vi "uA_Measurement_kit_v2.vi"() -> ()   [LabVIEW 2015]
uses:
  <vilib>/DAQmx/read.llb/DAQmx Read (Analog Wfm 1Chan NSamp).vi
  <vilib>/Utility/file.llb/Write Delimited Spreadsheet (string).vi
  <vilib>/measure/matone.llb/Extract Multiple Tone Information 1 Chan.vi
  <vilib>/DAQmx/miscellaneous.llb/DAQmx Fill In Error Info.vi
  <vilib>/measure/madcrms.llb/Basic Averaged DC-RMS for 1 Chan.vi
  <vilib>/measure/matone.llb/Extract Single Tone Information 1 Chan.vi
  <vilib>/measure/NI_MAPro.lvlib
  <vilib>/measure/NI_MABase.lvlib
panel:
  in  "uA_bank0":dbl=1.5 format="%#_13g"
  out "Task out":refnum<k21>="Stop"
  out "Sample rate":dbl=20000.0 format="%#_13g"
  out "Clear":bool=TRUE
  out "Ver":string
  out "seconds since 1Jan1904":timestamp
  out "error out":errorcluster
  in  "Tab Control":enum32{"Current Tracking", "Image", "CSV LOG"}(tab)
  out "uA_bank1":dbl
  in  "Calib":bool
  in  "Power ON/OFF":bool
  in  "Profile":enum16{"SAM", "DIANA", "Other..."}(ring)
  in  "Take Picture":bool
  in  "Orginal":bool
  in  "Clear Graph":bool
  out "Amp(Vdc)":dbl
  out "Freq(Hz)":dbl
  out "Waveform Graph 3":waveform(dbl)(graph)
  in  "ZOOM M1M2":bool
  in  "ZOOM -":bool
  in  "ZOOM +":bool
  in  "stop":bool
  out "VDUT- Vbat":dbl
  in  "Acquire Mode":enum16{"Streaming", "Read All", "Stop"}(ring)
  in  "Measure":bool
  in  "Current Range":T1(ring)
  out "Source":dbl
  in  "USB":tag="Dev1"
  out "Min value":dbl
  out "Max value":dbl
  out "Delta(s)":sgl
  in  "Center":bool
  out "Average":dbl
  in  "mA/uA":bool
  out "Waveform_main":waveform(sgl)(graph)
  out "Waveform_sub":waveform(dbl)(graph)
  out "Average (uA)":dbl
  in  "DUT Voltage Selector":enum16{"3.8VDC", "2.9VDC", "3.7VDC", "4.0VDC"}(ring)=enum."2.9VDC"
  in  "file List":i32(listbox)
  out "2D Picture":picture
  out "uA":dbl format="%#_4g"
  out "Vbat":dbl format="%#_4g"
  out "current time":timestamp
  in  "Record uA & Vbat":bool
  in  "Path":path
  out "uA":dbl(graph)
  out "Vbat Monitor":dbl(graph)
  # "uPower kit V2.1"
  # "Current"
  # "Voltage"
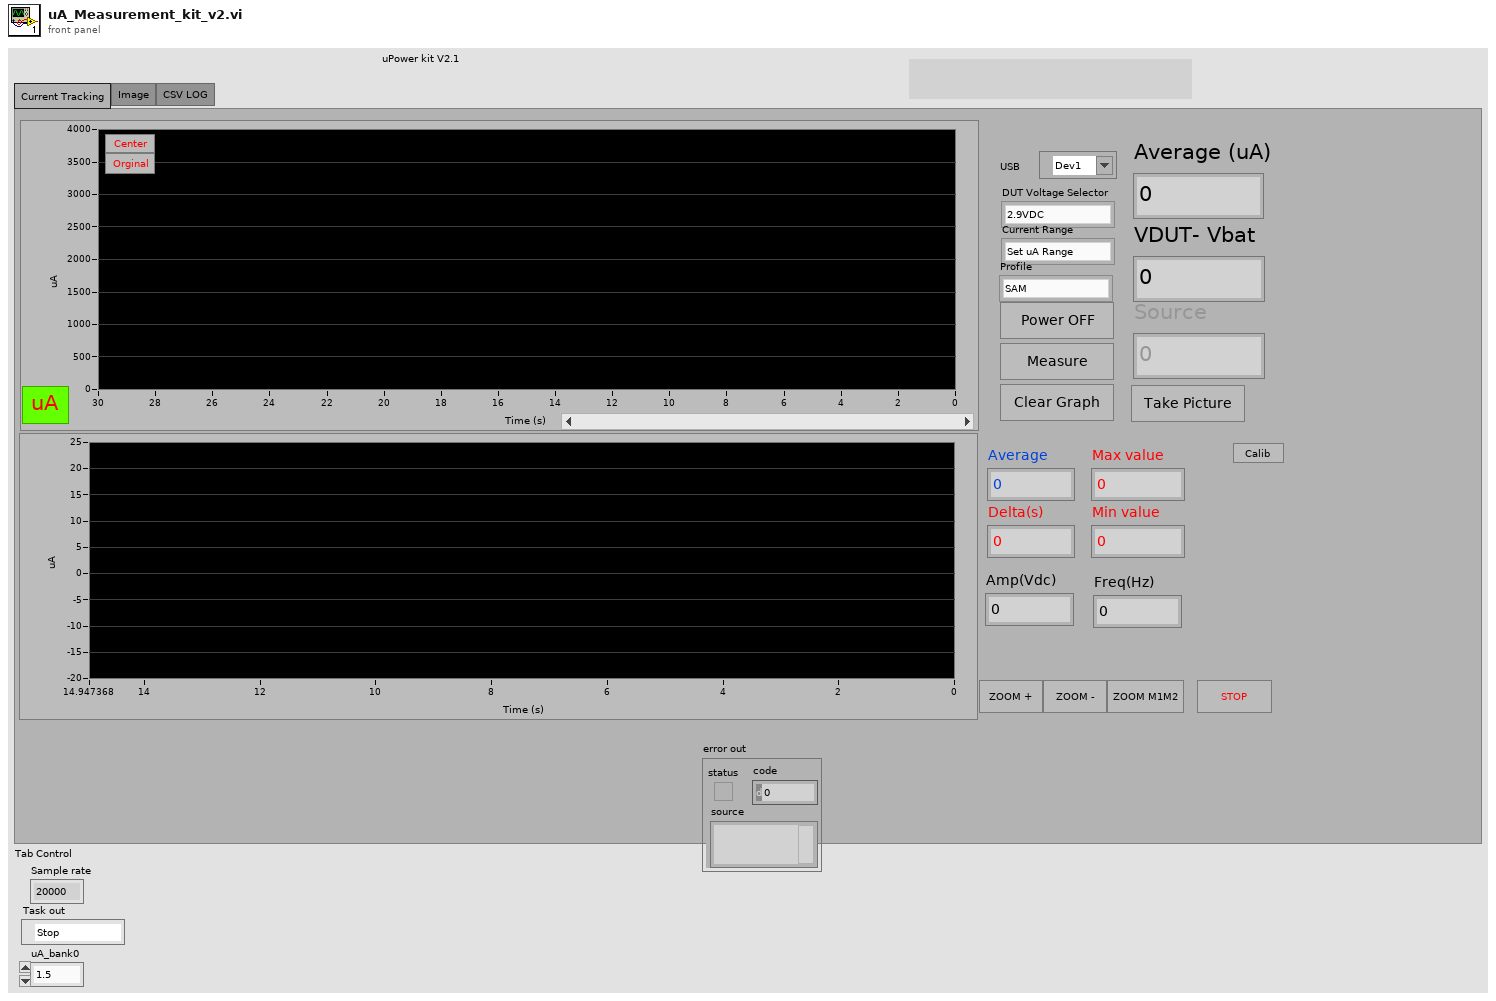
[diagram p1: front panel]
types:
  T1 = enum16{"Set uA Range ", "Set mA Range", "Measure Voltage"}
  T2 = typedef "LVCursorListTypeDef.ctl" = cluster{"Name":string, "Color":u32, "Style":u8, "Point Style":u8, "Name Visible":bool, "Allow Drag":bool, "Cursor Mode":u32, "Plot":i32, "Index":i32, "Position":cluster{"X":dbl, "Y":dbl}, "X Scale":u32, "Y Scale":u32, "Watch Plots":i32[], "Watch All Plots":bool, "Plot Area":i32, "Label Offset":cluster{"X":dbl, "Y":dbl}}[]
  T3 = typedef "imagedata.ctl" = cluster{"image type":i32, "image depth":i32, "image":u8[], "mask":u8[], "colors":u32[], "Rectangle":cluster{"left":i16, "top":i16, "right":i16, "bottom":i16}}
  T4 = enum32{"none", "input signal", "detected signal", "residual signal"}
  T5 = cluster{"detected frequency":dbl, "detected amplitude":dbl, "detected phase (deg)":dbl}[]
  T6 = cluster{"detected frequency":dbl, "detected amplitude":dbl, "detected phase (deg)":dbl}
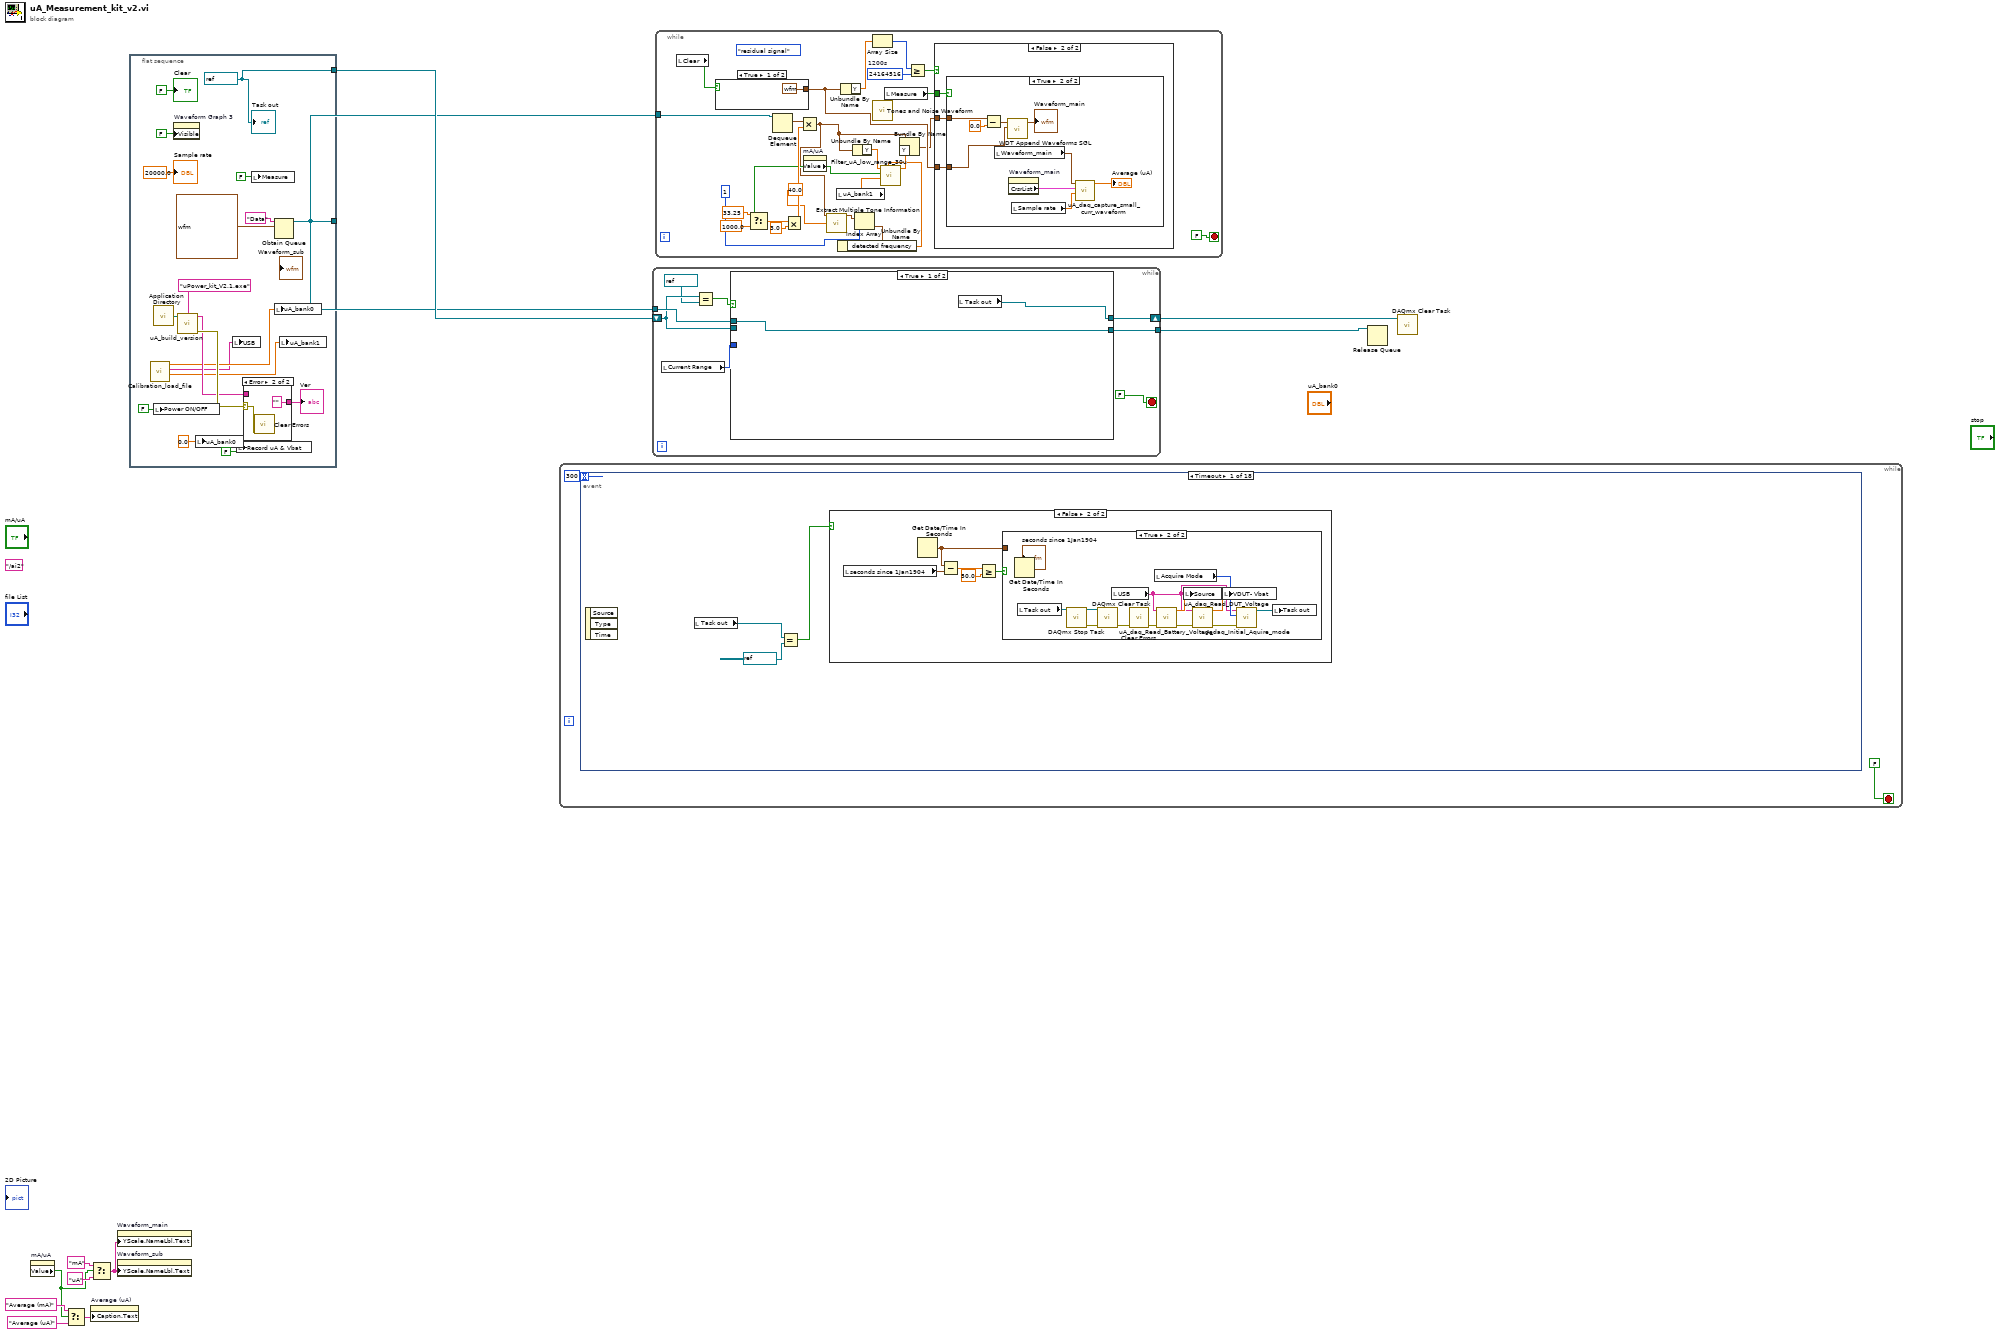
[diagram p0: block diagram]
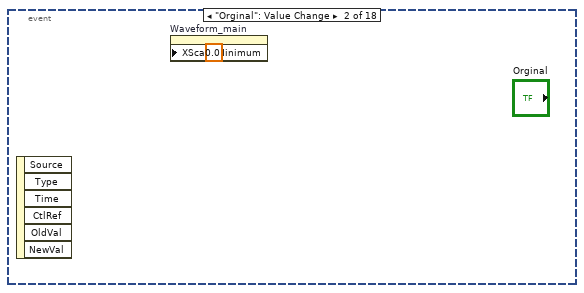
[diagram p5: hidden frame]
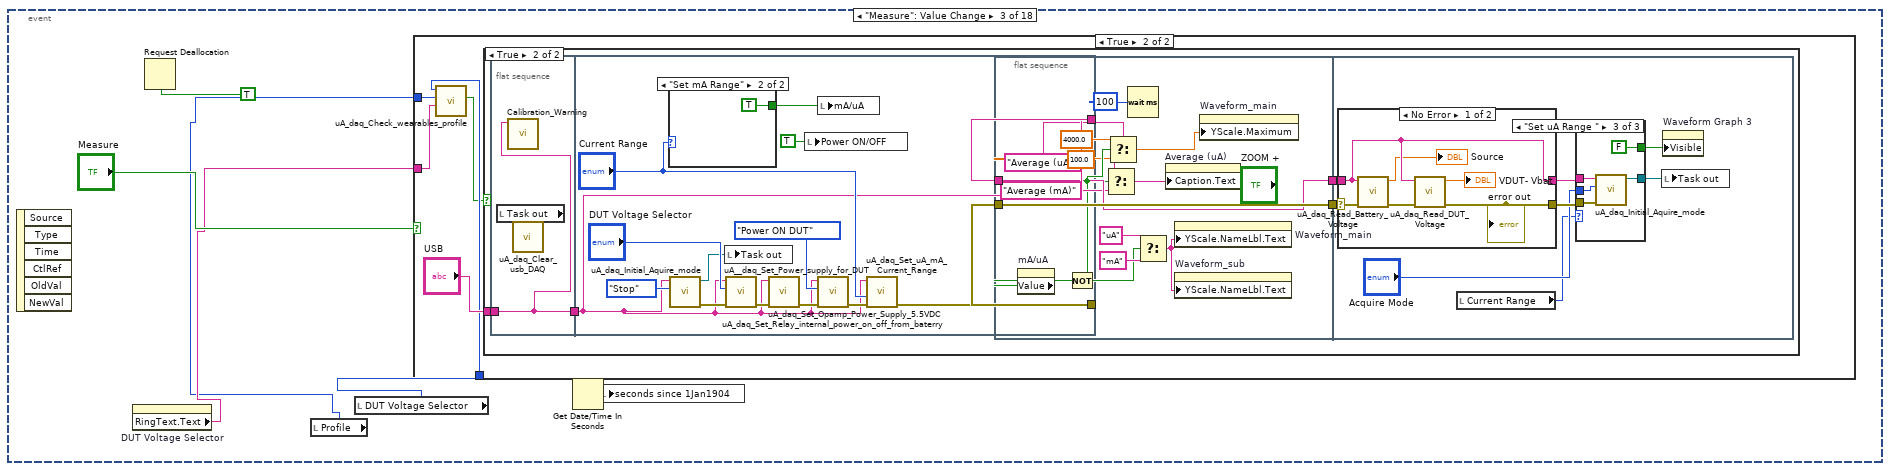
[diagram p6: hidden frame]
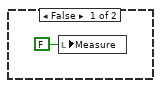
[diagram p8: hidden frame]
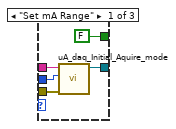
[diagram p9: hidden frame]
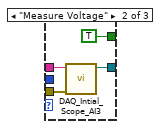
[diagram p10: hidden frame]
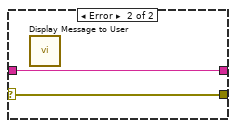
[diagram p11: hidden frame]
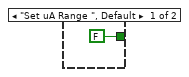
[diagram p12: hidden frame]
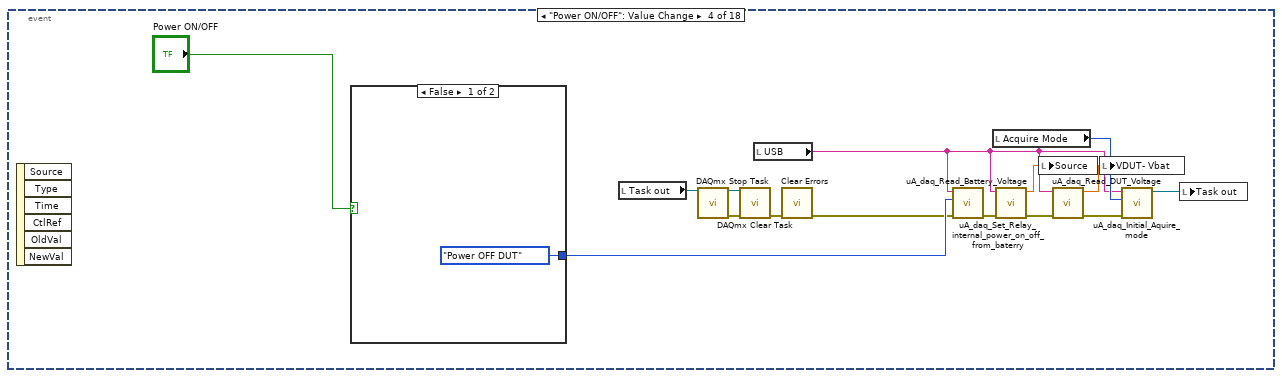
[diagram p13: hidden frame]
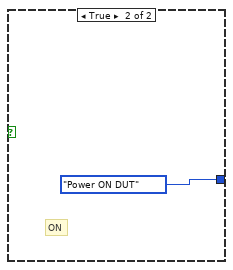
[diagram p14: hidden frame]
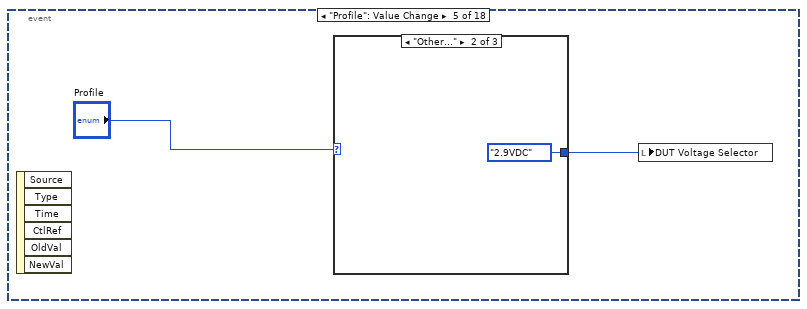
[diagram p15: hidden frame]
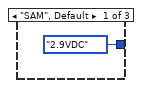
[diagram p16: hidden frame]
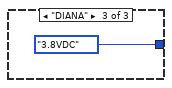
[diagram p17: hidden frame]
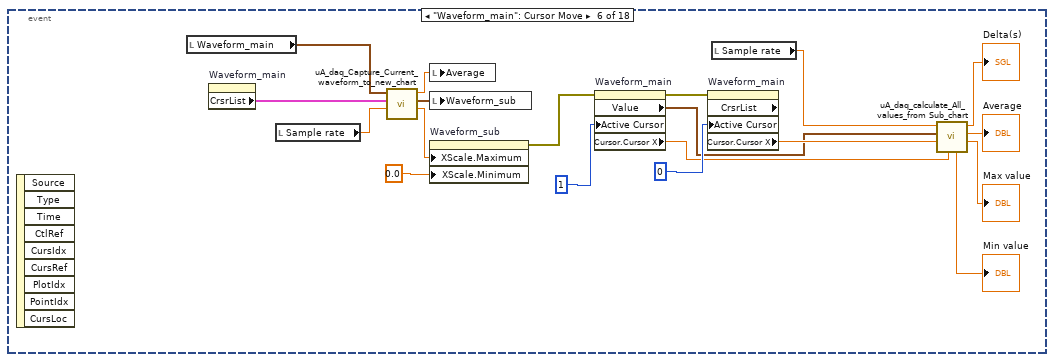
[diagram p18: hidden frame]
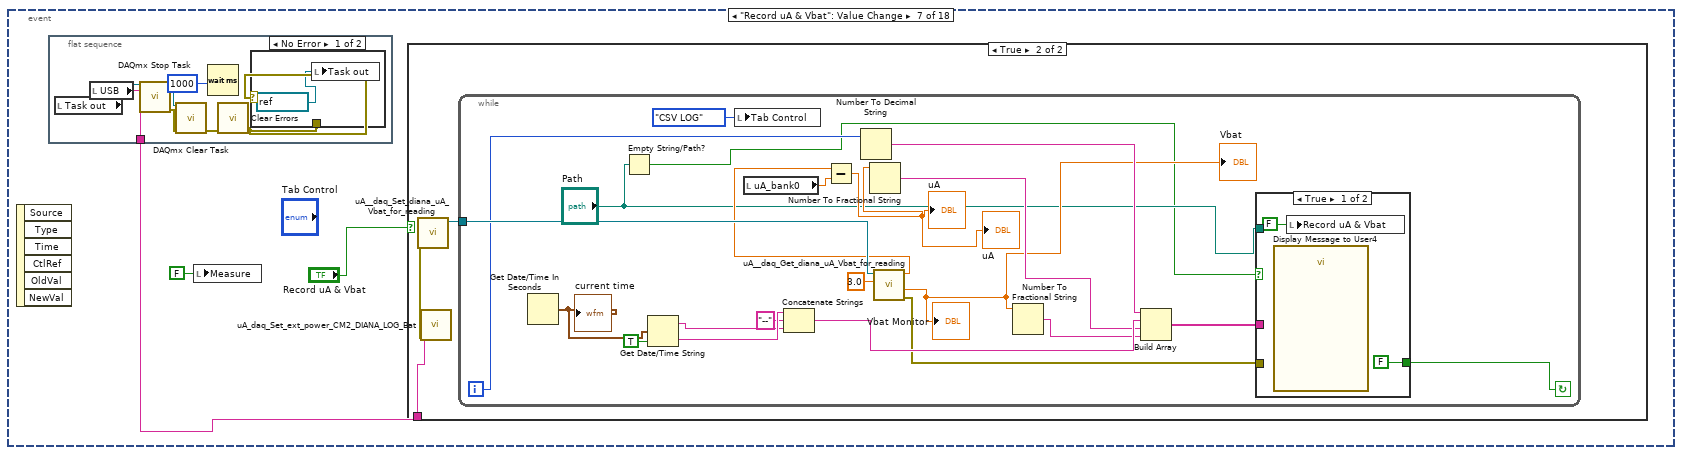
[diagram p19: hidden frame]
diagram:
  (unwired) "/ai2" ("string")
  n1 = property on="mA/uA" class="Bool (strict)"() -> ("Value"=w6:bool)  [unwired: 2 in, 2 out]
  n2 = Select(t="Average (mA)" ("Caption.Text"), s=w6, f="Average (uA)" ("Caption.Text")) -> (s? t:f=w4:string)
  n3 = property on="Average (uA)" class="DigNum (strict)"("Caption.Text"=w4) -> ()  [unwired: 2 in, 2 out]
  n4 = Select(t="mA" ("Caption.Text"), s=w6, f="uA" ("Caption.Text")) -> (s? t:f=w5:string)
  n5 = property on="Waveform_main" class="WFGraph (strict)"("YScale.NameLbl.Text"=w5) -> ()  [unwired: 2 in, 2 out]
  n6 = property on="Waveform_sub" class="WFGraph (strict)"("YScale.NameLbl.Text"=w5) -> ()  [unwired: 2 in, 2 out]
  n7 = flat-sequence {
    tunnel: [w22] -> w2
    tunnel: [w25] -> w1
    frame #0 {
      w22 = refnum<k21> "Stop" ("task out")
      n8 = call "Calibration_load_file.vi"() -> ("uABank1"=w15:dbl, "USB_DEV"=w14:string, "uABank0"=w16:dbl)  [unwired: 9 in]
      n9 = call <vilib>:"Application Directory.vi"() -> ("Application Directory"=w24:path)
      n10 = local write "Power ON/OFF"(FALSE ("Power ON/OFF")) -> ()
      n11 = property on="Waveform Graph 3" class="WFGraph (strict)"("Visible"=FALSE) -> ()  [unwired: 2 in, 2 out]
      n12 = call "uA_build_version.vi"("name or relative path"="uPower_kit_V2.1.exe", "path"=w24) -> ("error out"=w21:errorcluster, "FileVersion"=w20:string)  [unwired: 7 in, 1 out]
      n13 = local write "uA_bank0"(0.0 ("uA_calib_0")) -> ()
      n14 = local write "USB"(w14) -> ()
      n15 = local write "Record uA & Vbat"(FALSE ("Record uA & Vbat")) -> ()
      n16 = case shown="Error" w21 {
        selector: w21 -> [_ w33]
        tunnel: w20 -> [w31 _]
        tunnel: [w31 "" ("FileVersion")] -> w19
        frame No Error {
        }
        frame Error {
          n17 = call <vilib>:"Clear Errors.vi"("error in (no error)"=w33) -> ()  [unwired: 5 in, 2 out]
        }
      }
      "Ver" <- w19
      n18 = local write "Measure"(FALSE ("Measure")) -> ()
      n19 = Obtain Queue(name (unnamed)="Data", element data type=waveform(sgl) {"t0"=timestamp(0 s since 1904-01-01), "dt"=1.0, "Y"=[]} ("Waveform Chart 2")) -> (queue out=w25:refnum<queue>)  [unwired: 3 in, 2 out]
      n20 = local write "uA_bank0"(w16) -> ()
      n21 = local write "uA_bank1"(w15) -> ()
      "Clear" <- FALSE ("Clear")
      "Sample rate" <- 20000.0 ("Sample rate")
      "Task out" <- w22
    }
  }
  n22 = while {
    stop <- FALSE stop-if-true
    n23 = event shown="[0] Timeout" {
      selector: _ -> [_ _ _ _ _ _ _ _ _ _ _ _ _ _ _ _ _ _]
      dyn-events: _ -> [_ _ _ _ _ _ _ _ _ _ _ _ _ _ _ _ _ _]
      timeout: 300 -> [_ _ _ _ _ _ _ _ _ _ _ _ _ _ _ _ _ _]
      event Timeout {
        n24 = event-data() -> ()  [unwired: 1 in, 3 out]
        n25 = local read "Task out"() -> (w36:refnum<k21>)
        n26 = Equal?(x=w36, y=refnum<k21> "Stop") -> (x = y?=w37:bool)
        n27 = case shown="False" w37 {
          frame True {
          }
          frame False {
            n28 = local read "seconds since 1Jan1904"() -> (w39:timestamp)
            n29 = Get Date/Time In Seconds() -> (seconds since 1Jan1904=w40:timestamp)
            n30 = Subtract(x=w40, y=w39) -> (x-y=w43:dbl)
            n31 = Greater Or Equal?(x=w43, y=50.0) -> (x >= y?=w41:bool)
            n32 = case shown="True" w41 {
              tunnel: w40 -> [_ _]
              frame False {
              }
              frame True {
                n33 = Get Date/Time In Seconds() -> (seconds since 1Jan1904=→"seconds since 1Jan1904":timestamp)
                n34 = local read "Task out"() -> (w53:refnum<k21>)
                n35 = call <vilib>:"DAQmx Stop Task.vi"("task/channels in"=w53) -> ("task out"=w52:refnum<k21>, "error out"=w55:errorcluster)  [unwired: 13 in]
                n36 = call <vilib>:"DAQmx Clear Task.vi"("task in"=w52, "error in"=w55) -> ("error out"=w54:errorcluster)  [unwired: 13 in]
                n37 = local read "USB"() -> (w46:tag)
                n38 = call <vilib>:"Clear Errors.vi"("error in (no error)"=w54) -> ("error out"=w51:errorcluster)  [unwired: 5 in, 1 out]
                n39 = local read "Acquire Mode"() -> (w47:enum16{"Streaming", "Read All", "Stop"})
                n40 = call "uA_daq_Read_Battery_Voltage.vi"("error in"=w51, "USB DAQ"=w46) -> ("error out"=w48:errorcluster, "Battery_Voltage"=w50:dbl)  [unwired: 8 in]
                n41 = local write "Source"(w50) -> ()
                n42 = call "uA_daq_Read_DUT_Voltage.vi"("error in"=w48, "USB DAQ"=w46) -> ("error out"=w45:errorcluster, "DUT_Voltage"=w49:dbl)  [unwired: 8 in]
                n43 = local write "VDUT- Vbat"(w49) -> ()
                n44 = call "uA_daq_Initial_Aquire_mode.vi"("error in"=w45, "Acquire Mode"=w47, "USB DAQ"=w46) -> ("Refnum out"=w44:refnum<k21>)  [unwired: 7 in, 1 out]
                n45 = local write "Task out"(w44) -> ()
              }
            }
          }
        }
      }
      event "Orginal": Value Change {
        n46 = event-data() -> ()  [unwired: 1 in, 6 out]
        n47 = property on="Waveform_main" class="WFGraph (strict)"("XScale.Minimum"=0.0 ("X Scale.Range:Minimum")) -> ()  [unwired: 2 in, 2 out]
      }
      event "Measure": Value Change {
        n48 = event-data() -> ()  [unwired: 1 in, 6 out]
        n49 = property on="DUT Voltage Selector" class="Enum (strict)"() -> ("RingText.Text"=w60:string)  [unwired: 2 in, 2 out]
        n50 = Request Deallocation(TRUE ("flag")) -> ()
        n51 = local read "Profile"() -> (w58:enum16{"SAM", "DIANA", "Other..."})
        n52 = local read "DUT Voltage Selector"() -> (w59:enum16{"3.8VDC", "2.9VDC", "3.7VDC", "4.0VDC"})
        n53 = case shown="True" "Measure" {
          tunnel: w60 -> [_ w67]
          tunnel: w59 -> [_ w66]
          tunnel: w58 -> [_ w65]
          frame False {
          }
          frame True {
            n54 = call "uA_daq_Check_wearables_profile.vi"("VDUT"=w67, "Profile"=w65, "DUT Voltage Selector"=w66) -> ("Profile"=w64:bool)  [unwired: 7 in, 1 out]
            n55 = case shown="True" w64 {
              tunnel: "USB" -> [_ w71]
              frame False {
                n56 = local write "Measure"(FALSE ("Measure")) -> ()
              }
              frame True {
                n57 = flat-sequence {
                  tunnel: w71 -> [w120]
                  tunnel: [w120] -> w75
                  tunnel: [w129] -> w72
                  tunnel: [w123] -> w70
                  tunnel: w75 -> [w123]
                  frame #0 {
                    n58 = local read "Task out"() -> (w121:refnum<k21>)
                    n59 = call "Calibration_Warning.vi"("USB"=w120) -> ()  [unwired: 11 in]
                    n60 = call "uA_daq_Clear_usb_DAQ.vi"("Refnum in"=w121) -> ()  [unwired: 11 in]
                  }
                  frame #1 {
                    n61 = case shown="\"Set mA Range\"" "Current Range" {
                      tunnel: [FALSE ("mA/uA") TRUE ("mA/uA")] -> w127
                      frame "Set uA Range ", Default {
                      }
                      frame "Set mA Range" {
                      }
                    }
                    n62 = call "uA_daq_Initial_Aquire_mode.vi"("Acquire Mode"=enum16{"Streaming", "Read All", "Stop"}."Stop", "USB DAQ"=w123) -> ("error out"=w124:errorcluster, "Refnum out"=w125:refnum<k21>)  [unwired: 8 in]
                    n63 = local write "Task out"(w125) -> ()
                    n64 = call "uA__daq_Set_Power_supply_for_DUT.vi"("error in"=w124, "DUT Voltage Selector"="DUT Voltage Selector", "USB DAQ"=w123) -> ("error out"=w133:errorcluster)  [unwired: 8 in]
                    n65 = call "uA_daq_Set_Opamp_Power_Supply_5.5VDC.vi"("error in"=w133, "USB DAQ"=w123) -> ("error out"=w131:errorcluster)  [unwired: 9 in]
                    n66 = local write "Power ON/OFF"(TRUE ("Power ON/OFF")) -> ()
                    n67 = local write "mA/uA"(w127) -> ()
                    n68 = call "uA_daq_Set_Relay_internal_power_on_off_from_baterry.vi"("error in"=w131, "Power ON/OFF DUT"=enum16{"Power ON DUT", "Power OFF DUT"}."Power ON DUT", "USB DAQ"=w123) -> ("error out"=w130:errorcluster)  [unwired: 8 in]
                    n69 = call "uA_daq_Set_uA_mA_Current_Range.vi"("error in"=w130, "Current Range"="Current Range", "device name"=w123) -> ("error out"=w129:errorcluster)  [unwired: 8 in]
                  }
                }
                n70 = flat-sequence {
                  tunnel: w70 -> [w88]
                  tunnel: w72 -> [w89]
                  tunnel: [w89] -> w74
                  tunnel: [w88] -> w73
                  tunnel: w74 -> [w97]
                  tunnel: w73 -> [w96]
                  frame #0 {
                    n71 = property on="mA/uA" class="Bool (strict)"() -> ("Value"=w80:bool)  [unwired: 2 in, 2 out]
                    n72 = Not(x=w80) -> (.not. x?=w79:bool)
                    n73 = Select(t="Average (uA)" ("Caption.Text"), s=w79, f="Average (mA)" ("Caption.Text")) -> (s? t:f=w86:string)
                    n74 = Select(t=4000.0, s=w79, f=100.0) -> (s? t:f=w78:dbl)
                    n75 = Wait (ms)(milliseconds to wait=u32 100) -> ()  [unwired: 1 out]
                    n76 = Select(t="uA" ("Caption.Text"), s=w79, f="mA" ("Caption.Text")) -> (s? t:f=w81:string)
                    n77 = property on="Average (uA)" class="DigNum (strict)"("Caption.Text"=w86) -> ()  [unwired: 2 in, 2 out]
                    n78 = property on="Waveform_main" class="WFGraph (strict)"("YScale.NameLbl.Text"=w81) -> ()  [unwired: 2 in, 2 out]
                    n79 = property on="Waveform_sub" class="WFGraph (strict)"("YScale.NameLbl.Text"=w81) -> ()  [unwired: 2 in, 2 out]
                    n80 = property on="Waveform_main" class="WFGraph (strict)"("YScale.Maximum"=w78) -> ()  [unwired: 2 in, 2 out]
                  }
                  frame #1 {
                    n81 = case shown="No Error" w97 {
                      selector: w97 -> [w115 w119]
                      tunnel: w96 -> [w113 w118]
                      tunnel: [w114 w119] -> w95
                      tunnel: [w113 w118] -> w94
                      frame No Error {
                        n82 = call "uA_daq_Read_Battery_Voltage.vi"("error in"=w115, "USB DAQ"=w113) -> ("error out"=w117:errorcluster, "Battery_Voltage"=→"Source":dbl)  [unwired: 8 in]
                        n83 = call "uA_daq_Read_DUT_Voltage.vi"("error in"=w117, "USB DAQ"=w113) -> ("error out"=w114:errorcluster, "DUT_Voltage"=→"VDUT- Vbat":dbl)  [unwired: 8 in]
                        "error out" <- w114
                      }
                      frame Error {
                        n84 = call "Display Message to User"() -> ()  [unwired: 10 in, 2 out]
                      }
                    }
                    n85 = local read "Current Range"() -> (w91:T1)
                    n86 = case shown="\"Set uA Range \"" w91 {
                      tunnel: w95 -> [w102 w104 w111]
                      tunnel: w94 -> [w101 w106 w110]
                      tunnel: [w100 w105 w109] -> w93
                      tunnel: "Acquire Mode" -> [w99 _ w108]
                      tunnel: [FALSE ("Visible") TRUE ("Visible") FALSE ("Visible")] -> w90
                      frame "Set mA Range" {
                        n87 = call "uA_daq_Initial_Aquire_mode.vi"("error in"=w102, "Acquire Mode"=w99, "USB DAQ"=w101) -> ("Refnum out"=w100:refnum<k21>)  [unwired: 7 in, 1 out]
                      }
                      frame "Measure Voltage" {
                        n88 = call "DAQ_Intial_Scope_AI3.vi"("error in"=w104, "physical channel"=w106) -> ("task out"=w105:refnum<k21>)  [unwired: 8 in, 1 out]
                      }
                      frame "Set uA Range " {
                        n89 = call "uA_daq_Initial_Aquire_mode.vi"("error in"=w111, "Acquire Mode"=w108, "USB DAQ"=w110) -> ("Refnum out"=w109:refnum<k21>)  [unwired: 7 in, 1 out]
                      }
                    }
                    n90 = local write "Task out"(w93) -> ()
                    n91 = property on="Waveform Graph 3" class="WFGraph (strict)"("Visible"=w90) -> ()  [unwired: 2 in, 2 out]
                  }
                }
              }
            }
          }
        }
        n92 = Get Date/Time In Seconds() -> (seconds since 1Jan1904=w62:timestamp)
        n93 = local write "seconds since 1Jan1904"(w62) -> ()
      }
      event "Power ON/OFF": Value Change {
        n94 = event-data() -> ()  [unwired: 1 in, 6 out]
        n95 = case shown="False" "Power ON/OFF" {
          tunnel: [enum16{"Power ON DUT", "Power OFF DUT"}."Power OFF DUT" ("Power ON/OFF DUT") enum16{"Power ON DUT", "Power OFF DUT"}."Power ON DUT" ("Power ON/OFF DUT")] -> w141
          frame False {
          }
          frame True {
            # "ON"
          }
        }
        n96 = local read "Task out"() -> (w149:refnum<k21>)
        n97 = call <vilib>:"DAQmx Stop Task.vi"("task/channels in"=w149) -> ("task out"=w148:refnum<k21>, "error out"=w151:errorcluster)  [unwired: 13 in]
        n98 = call <vilib>:"DAQmx Clear Task.vi"("task in"=w148, "error in"=w151) -> ("error out"=w150:errorcluster)  [unwired: 13 in]
        n99 = local read "USB"() -> (w140:tag)
        n100 = call <vilib>:"Clear Errors.vi"("error in (no error)"=w150) -> ("error out"=w139:errorcluster)  [unwired: 5 in, 1 out]
        n101 = call "uA_daq_Set_Relay_internal_power_on_off_from_baterry.vi"("error in"=w139, "Power ON/OFF DUT"=w141, "USB DAQ"=w140) -> ("error out"=w138:errorcluster)  [unwired: 8 in]
        n102 = local read "Acquire Mode"() -> (w145:enum16{"Streaming", "Read All", "Stop"})
        n103 = call "uA_daq_Read_Battery_Voltage.vi"("error in"=w138, "USB DAQ"=w140) -> ("error out"=w137:errorcluster, "Battery_Voltage"=w147:dbl)  [unwired: 8 in]
        n104 = local write "Source"(w147) -> ()
        n105 = call "uA_daq_Read_DUT_Voltage.vi"("error in"=w137, "USB DAQ"=w140) -> ("error out"=w144:errorcluster, "DUT_Voltage"=w146:dbl)  [unwired: 8 in]
        n106 = local write "VDUT- Vbat"(w146) -> ()
        n107 = call "uA_daq_Initial_Aquire_mode.vi"("error in"=w144, "Acquire Mode"=w145, "USB DAQ"=w140) -> ("Refnum out"=w143:refnum<k21>)  [unwired: 7 in, 1 out]
        n108 = local write "Task out"(w143) -> ()
      }
      event "Profile": Value Change {
        n109 = event-data() -> ()  [unwired: 1 in, 6 out]
        n110 = case shown="\"Other...\"" "Profile" {
          tunnel: [enum16{"3.8VDC", "2.9VDC", "3.7VDC", "4.0VDC"}."2.9VDC" ("DUT Voltage Selector") enum16{"3.8VDC", "2.9VDC", "3.7VDC", "4.0VDC"}."2.9VDC" ("DUT Voltage Selector") enum16{"3.8VDC", "2.9VDC", "3.7VDC", "4.0VDC"}."3.8VDC" ("DUT Voltage Selector")] -> w154
          frame "SAM", Default {
          }
          frame "Other..." {
          }
          frame "DIANA" {
          }
        }
        n111 = local write "DUT Voltage Selector"(w154) -> ()
      }
      event "Waveform_main": Cursor Move {
        n112 = event-data() -> ()  [unwired: 1 in, 9 out]
        n113 = local read "Waveform_main"() -> (w167:waveform(sgl))
        n114 = property on="Waveform_main" class="WFGraph (strict)"() -> ("CrsrList"=w177:T2)  [unwired: 2 in, 2 out]
        n115 = local read "Sample rate"() -> (w166:dbl)
        n116 = call "uA_daq_Capture_Current_waveform_to_new_chart.vi"("Sample rate"=w166, "CrsrList"=w177, "Waveform_main"=w167) -> ("Numeric"=w174:dbl, "Waveform"=w175:waveform(sgl), "Numeric 2"=w176:sgl)  [unwired: 6 in]
        n117 = local write "Average"(w176) -> ()
        n118 = local write "Waveform_sub"(w175) -> ()
        n119 = property on="Waveform_sub" class="WFGraph (strict)"("XScale.Maximum"=w174, "XScale.Minimum"=0.0 ("X Scale.Range:Minimum")) -> (error out=w159:errorcluster)  [unwired: 2 in, 1 out]
        n120 = property on="Waveform_main" class="WFGraph (strict)"(error in=w159, "Active Cursor"=u32 1) -> (error out=w169:errorcluster, "Value"=w168:waveform(sgl), "Cursor.Cursor X"=w171:dbl)  [unwired: 1 in, 1 out]
        n121 = property on="Waveform_main" class="WFGraph (strict)" props=["CrsrList", "Active Cursor", "Cursor", "Cursor X"](error in=w169, "Active Cursor"=u32 0) -> ("Cursor.Cursor X"=w170:dbl)  [unwired: 1 in, 3 out]
        n122 = local read "Sample rate"() -> (w165:dbl)
        n123 = call "uA_daq_calculate_All_values_from Sub_chart.vi"("Cursor.Cursor X 2"=w171, "Cursor.Cursor X"=w170, "Value"=w168, "Sample rate"=w165) -> ("Max value"=→"Max value":dbl, "Average"=→"Average":dbl, "Delta(s)"=→"Delta(s)":sgl, "Min value"=→"Min value":dbl)  [unwired: 4 in]
      }
      event "Record uA & Vbat": Value Change {
        n124 = event-data() -> ()  [unwired: 1 in, 6 out]
        n125 = flat-sequence {
          tunnel: [w187] -> w179
          frame #0 {
            n126 = local read "Task out"() -> (w183:refnum<k21>)
            n127 = local read "USB"() -> (w187:tag)
            n128 = call <vilib>:"DAQmx Stop Task.vi"("task/channels in"=w183) -> ("task out"=w182:refnum<k21>, "error out"=w185:errorcluster)  [unwired: 13 in]
            n129 = call <vilib>:"DAQmx Clear Task.vi"("task in"=w182, "error in"=w185) -> ("error out"=w184:errorcluster)  [unwired: 13 in]
            n130 = Wait (ms)(milliseconds to wait=u32 1000) -> ()  [unwired: 1 out]
            n131 = call <vilib>:"Clear Errors.vi"("error in (no error)"=w184) -> ("error out"=w181:errorcluster)  [unwired: 5 in, 1 out]
            n132 = case shown="No Error" w181 {
              tunnel: w181 -> [_ _]
              frame No Error {
                n133 = local write "Task out"(refnum<k21> "Stop" ("y")) -> ()
              }
              frame Error {
              }
            }
          }
        }
        n134 = local write "Measure"(FALSE ("Measure")) -> ()
        n135 = case shown="True" "Record uA & Vbat" {
          tunnel: w179 -> [_ w191]
          frame False {
          }
          frame True {
            n136 = call "uA_daq_Set_ext_power_CM2_DIANA_LOG_Bat.vi"("USB DAQ in"=w191) -> ("error out"=w192:errorcluster, "USB DAQ out"=w190:tag)  [unwired: 9 in]
            n137 = call "uA__daq_Set_diana_uA_Vbat_for_reading.vi"("error in (no error)"=w192, "USB DAQ in"=w190) -> ("Refnum out"=w189:refnum<k21>)  [unwired: 8 in, 1 out]
            n138 = while {
              tunnel: w189 -> [w214]
              i -> [w204]
              stop <- w193 continue-if-true
              n139 = Get Date/Time In Seconds() -> (seconds since 1Jan1904=w213:timestamp)
              "current time" <- w213
              n140 = Empty String/Path?(string/path="Path") -> (empty?=w194:bool)
              n141 = Get Date/Time String(seconds (now)=w213, want seconds? (F)=TRUE) -> (date string=w211:string, time string=w212:string)  [unwired: 1 in]
              n142 = local write "Tab Control"(enum32{"Current Tracking", "Image", "CSV LOG"}."CSV LOG" ("Tab Control")) -> ()
              n143 = local read "uA_bank0"() -> (w199:dbl)
              n144 = Concatenate Strings(w212, "--" ("string"), w211) -> (w209:string)
              n145 = Number To Decimal String(number=w204) -> (decimal integer string=w203:string)  [unwired: 1 in]
              n146 = call "uA__daq_Get_diana_uA_Vbat_for_reading.vi"("Coef"=3.0, "Refnum in"=w214) -> ("error out"=w200:errorcluster, "Vbat"=w202:dbl, "uA Current"=w198:dbl)  [unwired: 5 in, 2 out]
              "Vbat Monitor" <- w202
              "Vbat" <- w202
              n147 = Subtract(x=w198, y=w199) -> (x-y=w197:dbl)
              "uA" <- w197
              "uA" <- w197
              n148 = Number To Fractional String(number=w197) -> (F-format string=w208:string)  [unwired: 3 in]
              n149 = Number To Fractional String(number=w202) -> (F-format string=w207:string)  [unwired: 3 in]
              n150 = Build Array(w203, w209, w208, w207) -> (w206:string[])
              n151 = case shown="True" w194 {
                tunnel: w206 -> [_ w220]
                tunnel: w200 -> [_ w219]
                tunnel: "Path" -> [_ w218]
                tunnel: [FALSE ("Record uA & Vbat") w217] -> w193
                frame True {
                  n152 = call "Display Message to User4"() -> ()  [unwired: 10 in, 2 out]
                  n153 = local write "Record uA & Vbat"(FALSE ("Record uA & Vbat")) -> ()
                }
                frame False {
                  n154 = local read "Record uA & Vbat"() -> (w217:bool)
                  n155 = case shown="No Error" w219 {
                    tunnel: w220 -> [w224 _]
                    tunnel: w218 -> [w221 _]
                    frame No Error {
                      n156 = call-poly <vilib>:"Write Delimited Spreadsheet.vi"("file path (dialog if empty)"=w221, "1D data"=w224, "append to file? (F)"=TRUE, "delimiter (\\t)"=";" ("delimiter (\\t)")) -> ()  [unwired: 10 in, 2 out]
                    }
                    frame Error {
                    }
                  }
                }
              }
            }
          }
        }
      }
      event "Calib": Value Change {
        n157 = event-data() -> ()  [unwired: 1 in, 6 out]
        n158 = property on="mA/uA" class="Bool (strict)"() -> ("Value"=w227:bool)  [unwired: 2 in, 2 out]
        n159 = case shown="False" w227 {
          tunnel: [w228 _] -> w225
          frame False {
            w235 = 3.0  # Coef 10Ohm:3
            # "uA"
            n160 = flat-sequence {
              tunnel: [w244] -> w233
              frame #0 {
                n161 = call "Display Message to User2"() -> ()  [unwired: 10 in, 2 out]
                n162 = local write "Measure"(FALSE ("Measure")) -> ()
              }
              frame #1 {
                n163 = local read "Task out"() -> (w241:refnum<k21>)
                n164 = Wait (ms)(milliseconds to wait=u32 1000) -> ()  [unwired: 1 out]
                n165 = call <vilib>:"DAQmx Stop Task.vi"("task/channels in"=w241) -> ("task out"=w240:refnum<k21>, "error out"=w242:errorcluster)  [unwired: 13 in]
                n166 = call <vilib>:"DAQmx Clear Task.vi"("task in"=w240, "error in"=w242) -> ("error out"=w239:errorcluster)  [unwired: 13 in]
                n167 = case shown="No Error" w239 {
                  frame No Error {
                    n168 = local write "Task out"(refnum<k21> "Stop" ("y")) -> ()
                  }
                  frame Error {
                  }
                }
                n169 = local read "USB"() -> (w244:tag)
              }
            }
            n170 = call "uA_daq_Set_ext_power_CM2_DIANA_LOG_Bat.vi"("USB DAQ in"=w233) -> ("error out"=w230:errorcluster, "USB DAQ out"=w237:tag)  [unwired: 9 in]
            n171 = call "uA__daq_Set_diana_uA_Vbat_for_reading.vi"("error in (no error)"=w230, "USB DAQ in"=w237) -> ("error out"=w231:errorcluster, "Refnum out"=w236:refnum<k21>)  [unwired: 8 in]
            n172 = call "uA__daq_Get_diana_uA_Vbat_for_reading.vi"("error in (no error)"=w231, "Coef"=w235, "Refnum in"=w236) -> ("error out"=w232:errorcluster, "uA Current"=w234:dbl)  [unwired: 4 in, 3 out]
            n173 = local write "uA_bank0"(w234) -> ()
            n174 = call "Calibration_Read_streaming_3s.vi"("error in (no error)"=w232, "USB"=w233) -> ("error out"=w228:errorcluster, "uABank1"=w229:dbl)  [unwired: 8 in]
            "uA_bank1" <- w229
            n175 = call "Calibration_Save_file.vi"("USB_DEV"=w233, "uABank1"=w229, "uABank0"=w234) -> ()  [unwired: 9 in]
          }
          frame True {
            # "mA"
          }
        }
        n176 = call "Display Message to User3"("error in (no error)"=w225, "Enable"=TRUE) -> ()  [unwired: 8 in, 2 out]
      }
      event "Clear Graph": Value Change {
        n177 = event-data() -> ()  [unwired: 1 in, 6 out]
        n178 = flat-sequence {
          frame #0 {
            w246 = waveform(sgl) {"t0"=timestamp(0 s since 1904-01-01), "dt"=1.0, "Y"=[]} ("Waveform_main")
            n179 = local write "Waveform_main"(w246) -> ()
            n180 = local write "Clear"(TRUE ("Clear")) -> ()
            n181 = Wait (ms)(milliseconds to wait=u32 500) -> ()  [unwired: 1 out]
            n182 = local write "Waveform_sub"(w246) -> ()
          }
          frame #1 {
            n183 = local write "Clear"(FALSE ("Clear")) -> ()
          }
        }
      }
      event "ZOOM +": Value Change {
        n184 = event-data() -> ()  [unwired: 1 in, 6 out]
        n185 = property on="Waveform_main" class="WFGraph (strict)" props=["XScale", "Range", "XScale", "Increment", "XScale", "Maximum", "XScale", "Minimum"]() -> ("XScale.Maximum"=w255:dbl, "XScale.Minimum"=w251:dbl)  [unwired: 2 in, 4 out]
        n186 = Subtract(x=w255, y=0.1) -> (x-y=w253:dbl)
        n187 = Add(x=w251, y=0.1) -> (x+y=w250:dbl)
        n188 = property on="Waveform_main" class="WFGraph (strict)"("XScale.Maximum"=w253, "XScale.Minimum"=w250) -> ()  [unwired: 2 in, 2 out]
      }
      event "ZOOM -": Value Change {
        n189 = event-data() -> ()  [unwired: 1 in, 6 out]
        n190 = property on="Waveform_main" class="WFGraph (strict)" props=["XScale", "Range", "XScale", "Increment", "XScale", "Maximum", "XScale", "Minimum"]() -> ("XScale.Maximum"=w264:dbl, "XScale.Minimum"=w260:dbl)  [unwired: 2 in, 4 out]
        n191 = Subtract(x=w260, y=0.1) -> (x-y=w257:dbl)
        n192 = Less Than 0?(x=w257) -> (x < 0?=w259:bool)
        n193 = Add(x=w264, y=0.1) -> (x+y=w262:dbl)
        n194 = Select(t=0.0, s=w259, f=w257) -> (s? t:f=w256:dbl)
        n195 = property on="Waveform_main" class="WFGraph (strict)"("XScale.Maximum"=w262, "XScale.Minimum"=w256) -> ()  [unwired: 2 in, 2 out]
      }
      event "ZOOM M1M2": Value Change {
        n196 = event-data() -> ()  [unwired: 1 in, 6 out]
        n197 = property on="Waveform_main" class="WFGraph (strict)"("Active Cursor"=u32 0) -> (error out=w271:errorcluster)  [unwired: 2 in, 1 out]
        n198 = property on="Waveform_main" class="WFGraph (strict)"(error in=w271) -> (error out=w268:errorcluster, "Cursor.Cursor X"=w266:dbl)  [unwired: 1 in, 1 out]
        n199 = property on="Waveform_main" class="WFGraph (strict)"(error in=w268, "Active Cursor"=u32 1) -> (error out=w270:errorcluster)  [unwired: 1 in, 1 out]
        n200 = property on="Waveform_main" class="WFGraph (strict)"(error in=w270) -> ("Cursor.Cursor X"=w265:dbl)  [unwired: 1 in, 2 out]
        n201 = Greater?(x=w266, y=w265) -> (0:w267:bool)
        n202 = case shown="True" w267 {
          tunnel: w266 -> [w274 w276]
          tunnel: w265 -> [w273 w275]
          frame False {
            n203 = property on="Waveform_main" class="WFGraph (strict)"("XScale.Maximum"=w273, "XScale.Minimum"=w274) -> ()  [unwired: 2 in, 2 out]
          }
          frame True {
            n204 = property on="Waveform_main" class="WFGraph (strict)"("XScale.Maximum"=w276, "XScale.Minimum"=w275) -> ()  [unwired: 2 in, 2 out]
          }
        }
      }
      event "Waveform_main": Mouse Down {
        n205 = event-data() -> ()  [unwired: 1 in, 8 out]
      }
      event "Tab Control": Value Change {
        n206 = event-data() -> ()  [unwired: 1 in, 6 out]
        n207 = call <vilib>:"Application Directory.vi"() -> ("Application Directory"=w279:path)
        n208 = call <userlib>:"List Directory__ogtk.vi"("pattern"="*.bmp", "directory path"=w279) -> ("file names"=w277:string[])  [unwired: 2 in, 3 out]
        n209 = property on="file List" class="LstBox (strict)"("Item Names"=w277) -> ()  [unwired: 2 in, 2 out]
      }
      event "Center": Value Change {
        n210 = event-data() -> ()  [unwired: 1 in, 6 out]
        n211 = property on="Waveform_main" class="WFGraph (strict)"() -> ("XScale.Maximum"=w284:dbl, "XScale.Minimum"=w283:dbl)  [unwired: 2 in, 2 out]
        n212 = Add(x=w284, y=w283) -> (x+y=w282:dbl)
        n213 = Divide(x=w282, y=2.0) -> (x/y=w280:dbl)
        n214 = property on="Waveform_main" class="WFGraph (strict)" props=["Value", "Active Cursor", "Cursor", "Cursor X"]("Active Cursor"=u32 1, "Cursor.Cursor X"=w280) -> (error out=w285:errorcluster)  [unwired: 2 in, 2 out]
        n215 = property on="Waveform_main" class="WFGraph (strict)" props=["CrsrList", "Active Cursor", "Cursor", "Cursor X"](error in=w285, "Active Cursor"=u32 0, "Cursor.Cursor X"=w280) -> ()  [unwired: 1 in, 3 out]
      }
      event "stop": Value Change {
        n216 = event-data() -> ()  [unwired: 1 in, 6 out]
        n217 = flat-sequence {
          frame #0 {
            n218 = local read "Task out"() -> (w289:refnum<k21>)
            n219 = call <vilib>:"DAQmx Stop Task.vi"("task/channels in"=w289) -> ("task out"=w288:refnum<k21>, "error out"=w291:errorcluster)  [unwired: 13 in]
            n220 = call <vilib>:"DAQmx Clear Task.vi"("task in"=w288, "error in"=w291) -> ("error out"=w290:errorcluster)  [unwired: 13 in]
            n221 = call <vilib>:"Clear Errors.vi"("error in (no error)"=w290) -> ()  [unwired: 5 in, 2 out]
          }
          frame #1 {
            n222 = local read "USB"() -> (w295:tag)
            n223 = call "uA_daq_Set_Relay_internal_power_on_off_from_baterry.vi"("Power ON/OFF DUT"=enum16{"Power ON DUT", "Power OFF DUT"}."Power OFF DUT", "USB DAQ"=w295) -> ("error out"=w294:errorcluster)  [unwired: 9 in]
            n224 = call "uA_daq_Set_Opamp_Power_Supply_Zero_voltageVDC.vi"("error in"=w294, "USB DAQ"=w295) -> ("error out"=w292:errorcluster)  [unwired: 9 in]
            n225 = call <vilib>:"Clear Errors.vi"("error in (no error)"=w292) -> ()  [unwired: 5 in, 2 out]
          }
          frame #2 {
            n226 = local read "Ver"() -> (w296:string)
            n227 = Empty String/Path?(string/path=w296) -> (empty?=w297:bool)
            n228 = case shown="True" w297 {
              frame True {
              }
              frame False {
                n229 = Quit LabVIEW(quit? (T)=TRUE) -> ()
              }
            }
          }
          frame #3 {
            n230 = Stop(stop? (T)=TRUE) -> ()
          }
        }
      }
      event "file List": Value Change {
        n231 = event-data() -> ()  [unwired: 1 in, 6 out]
        n232 = property on="file List" class="LstBox (strict)"() -> ("Value"=w306:i32, "Item Names"=w307:string[])  [unwired: 2 in, 2 out]
        n233 = Index Array(array=w307, index=w306) -> (element=w302:string)
        n234 = call <vilib>:"Application Directory.vi"() -> ("Application Directory"=w303:path)
        n235 = Build Path(base path=w303, name or relative path=w302) -> (appended path=w301:path)
        n236 = call <vilib>:"Read BMP File.vi"("path to BMP file"=w301) -> ("image data"=w305:T3)  [unwired: 8 in, 2 out]
        n237 = call <vilib>:"Draw Flattened Pixmap.vi"("image data"=w305) -> ("new picture"=w304:picture)  [unwired: 8 in]
        n238 = property on="2D Picture" class="Pict"("Value"=w304, "ZoomFactor"=sgl 0.75 ("Zoom Factor")) -> ()  [unwired: 2 in, 2 out]
      }
      event "Take Picture": Value Change {
        n239 = event-data() -> ()  [unwired: 1 in, 6 out]
        n240 = call <vilib>:"Application Directory.vi"() -> ("Application Directory"=w309:path)
        n241 = call "File Dialog2"("start path"=w309, "pattern (all files)"="*.bmp", "pattern label"="*.bmp") -> ("selected path"=w315:path, "error out"=w312:errorcluster)  [unwired: 9 in, 2 out]
        n242 = control-ref of="This VI"() -> (w313:refnum<vi>)
        n243 = invoke on="Invoke Node" class="VI" method="FP.Get Image"(reference=w313, "image depth"=enum32{"File", "Clipboard"}."File" ("Target")) -> ("image data"=w314:T3)  [unwired: 4 in, 5 out]
        n244 = call <vilib>:"Clear Errors.vi"("error in (no error)"=w312) -> ()  [unwired: 5 in, 2 out]
        n245 = call <vilib>:"Write BMP File.vi"("image data"=w314, "path to BMP file"=w315) -> ()  [unwired: 8 in, 2 out]
      }
    }
  }
  n246 = while {
    tunnel: w1 -> [w323]
    tunnel: [w322] -> w11
    shift-right: [w318] -> w3
    shift-left: w2 -> [w320]
    stop <- FALSE ("stop (F)") stop-if-true
    n247 = local read "Current Range"() -> (w317:T1)
    n248 = Equal?(x=w320, y=refnum<k21> "Stop") -> (x = y?=w316:bool)
    n249 = case shown="True" w316 {
      tunnel: w323 -> [w325 w330]
      tunnel: [w325 w329] -> w322
      tunnel: w320 -> [_ w328]
      tunnel: [w324 w327] -> w318
      tunnel: w317 -> [_ w326]
      frame True {
        n250 = local read "Task out"() -> (w324:refnum<k21>)
      }
      frame False {
        n251 = case shown="\"Set uA Range \"" w326 {
          tunnel: w330 -> [w341 w346 w368]
          tunnel: [w340 w346 w367] -> w329
          tunnel: w328 -> [w339 w357 w366]
          tunnel: [w338 w356 w365] -> w327
          frame "Set mA Range" {
            w337 = 10.0  # timeout (s)
            n252 = call-poly <vilib>:"DAQmx Read.vi"("task/channels in"=w339, "number of samples per channel"=10000, "timeout"=w337) -> ("data"=w332:waveform(dbl), "error out"=w335:errorcluster)  [unwired: 10 in, 1 out]
            n253 = Unbundle By Name(w332) -> ("Y"=w334:dbl[])
            n254 = Reverse 1D Array(array=w334) -> (reversed array=w331:dbl[])
            n255 = Bundle By Name(cluster=w332, "Y"=w331) -> (w333:waveform(dbl))
            n256 = case shown="No Error" w335 {
              selector: w335 -> [_ w345]
              tunnel: w341 -> [w344 _]
              tunnel: [w343 _] -> w340
              tunnel: w333 -> [w342 _]
              frame No Error {
                n257 = Enqueue Element(queue=w344, element=w342) -> (queue out=w343:refnum<queue>)  [unwired: 2 in, 2 out]
              }
              frame Error {
                n258 = call <vilib>:"Clear Errors.vi"("error in (no error)"=w345) -> ()  [unwired: 5 in, 2 out]
              }
            }
            n259 = local read "Task out"() -> (w338:refnum<k21>)
          }
          frame "Measure Voltage" {
            w355 = 10.0  # timeout (s)
            n260 = call-poly <vilib>:"DAQmx Read.vi"("task/channels in"=w357, "number of samples per channel"=5000, "timeout"=w355) -> ("data"=w350:waveform(dbl), "error out"=w353:errorcluster)  [unwired: 10 in, 1 out]
            "Waveform Graph 3" <- w350
            n261 = call <vilib>:"Clear Errors.vi"("error in (no error)"=w353) -> ()  [unwired: 5 in, 2 out]
            n262 = call-poly <vilib>:"Basic Averaged DC-RMS.vi"("averaging type"=enum16{"Linear", "Exponential"}."Linear", "signal in"=w350) -> ("error out"=w347:errorcluster, "DC value"=→"Amp(Vdc)":dbl)  [unwired: 6 in, 2 out]
            n263 = call-poly <vilib>:"Extract Single Tone Information.vi"("time signal in"=w350) -> ("error out"=w351:errorcluster, "detected frequency"=→"Freq(Hz)":dbl)  [unwired: 5 in, 4 out]
            n264 = local read "Task out"() -> (w356:refnum<k21>)
            n265 = call <vilib>:"Clear Errors.vi"("error in (no error)"=w351) -> ()  [unwired: 5 in, 2 out]
            n266 = call <vilib>:"Clear Errors.vi"("error in (no error)"=w347) -> ()  [unwired: 5 in, 2 out]
          }
          frame "Set uA Range " {
            w364 = 10.0  # timeout (s)
            n267 = call-poly <vilib>:"DAQmx Read.vi"("task/channels in"=w366, "number of samples per channel"=10000, "timeout"=w364) -> ("data"=w359:waveform(dbl), "error out"=w362:errorcluster)  [unwired: 10 in, 1 out]
            n268 = Unbundle By Name(w359) -> ("Y"=w361:dbl[])
            n269 = Reverse 1D Array(array=w361) -> (reversed array=w358:dbl[])
            n270 = Bundle By Name(cluster=w359, "Y"=w358) -> (w360:waveform(dbl))
            n271 = case shown="Error" w362 {
              selector: w362 -> [_ w372]
              tunnel: w368 -> [w371 _]
              tunnel: [w370 _] -> w367
              tunnel: w360 -> [w369 _]
              frame No Error {
                n272 = Enqueue Element(queue=w371, element=w369) -> (queue out=w370:refnum<queue>)  [unwired: 2 in, 2 out]
              }
              frame Error {
                n273 = call <vilib>:"Clear Errors.vi"("error in (no error)"=w372) -> ()  [unwired: 5 in, 2 out]
              }
            }
            n274 = local read "Task out"() -> (w365:refnum<k21>)
          }
        }
      }
    }
  }
  n275 = while {
    tunnel: w1 -> [w394]
    stop <- FALSE stop-if-true
    (unwired) T4."residual signal" ("export mode")
    w387 = 24164516  # 1200s
    n276 = local read "Clear"() -> (w392:bool)
    n277 = case shown="True" w392 {
      tunnel: [waveform(sgl) {"t0"=timestamp(0 s since 1904-01-01), "dt"=1.0, "Y"=[]} ("Waveform_main") w413] -> w391
      frame True {
      }
      frame False {
        n278 = local read "Waveform_main"() -> (w413:waveform(sgl))
      }
    }
    n279 = Dequeue Element(queue=w394) -> (element=w393:waveform(sgl))  [unwired: 2 in, 3 out]
    n280 = property on="mA/uA" class="Bool (strict)"() -> ("Value"=w380:bool)  [unwired: 2 in, 2 out]
    n281 = Select(t=sgl 33.25 ("y"), s=w380, f=sgl 1000.0 ("y")) -> (s? t:f=w386:sgl)
    n282 = Multiply(x=w386, y=sgl 3.0) -> (x*y=w385:sgl)
    n283 = Multiply(x=w393, y=w385) -> (x*y=w378:waveform(sgl))
    n284 = call-poly <vilib>:"Extract Multiple Tone Information.vi"("time signal in"=w378, "threshold"=40.0 ("Numeric 2")) -> ("multiple tone information"=w377:T5)  [unwired: 11 in, 2 out]
    n285 = local read "uA_bank1"() -> (w379:dbl)
    n286 = Unbundle By Name(w391) -> ("Y"=w390:sgl[])
    n287 = Unbundle By Name(w378) -> ("Y"=w382:sgl[])
    n288 = Index Array(array=w377, index=u16 1 ("Index")) -> (element=w376:T6)
    n289 = Unbundle By Name(w376) -> ("detected frequency"=w373:dbl)
    n290 = Array Size(array=w390) -> (size(s)=w397:i32)
    n291 = call <vilib>:"Tones and Noise Waveform.vi"() -> ()  [unwired: 10 in, 2 out]
    n292 = call "Filter_uA_low_range_30u.vi"("Frequency"=w373, "uA_calib_0"=w379, "mA/uA"=w380, "in"=w382) -> ("out"=w381:dbl[])  [unwired: 7 in]
    n293 = local read "Measure"() -> (w389:bool)
    n294 = Bundle By Name(cluster=w378, "Y"=w381) -> (w383:waveform(sgl))
    n295 = Greater Or Equal?(x=w397, y=w387) -> (x >= y?=w388:bool)
    n296 = case shown="False" w388 {
      tunnel: w383 -> [_ w402]
      tunnel: w391 -> [_ w401]
      tunnel: w389 -> [_ w400]
      frame True {
        n297 = local write "Measure"(FALSE ("Measure")) -> ()
      }
      frame False {
        n298 = case shown="True" w400 {
          tunnel: w402 -> [_ w410]
          tunnel: w401 -> [_ w403]
          frame False {
          }
          frame True {
            n299 = Subtract(x=w410, y=sgl 0.0) -> (x-y=w404:waveform(sgl))
            n300 = local read "Waveform_main"() -> (w407:waveform(sgl))
            n301 = call "WDT Append Waveforms SGL.vi"("waveform B"=w403, "waveform A"=w404) -> ("waveform out"=→"Waveform_main":waveform(sgl))  [unwired: 8 in, 1 out]
            n302 = property on="Waveform_main" class="WFGraph (strict)"() -> ("CrsrList"=w408:T2)  [unwired: 2 in, 2 out]
            n303 = local read "Sample rate"() -> (w406:dbl)
            n304 = call "uA_daq_capture_small_curr_waveform.vi"("Sample rate"=w406, "CrsrList"=w408, "Waveform_main"=w407) -> ("Numeric"=→"Average (uA)":sgl)  [unwired: 8 in]
          }
        }
      }
    }
  }
  n305 = Release Queue(queue=w11) -> ()  [unwired: 2 in, 3 out]
  n306 = call <vilib>:"DAQmx Clear Task.vi"("task in"=w3) -> ()  [unwired: 14 in, 1 out]
